vi "RegisterMessageQue.vi"(8 "error in (no error)":errorcluster, 9 "Message que":T1, 11 "SendMessage in":refnum<class "SendMessage.lvclass">) -> (0 "error out":errorcluster, 3 "SendMessage out":refnum<class "SendMessage.lvclass">)   [LabVIEW 2018, in "SendMessage.lvclass"]
uses:
  SendMessage.lvclass
  Support/MessageQue/MessageQue.ctl
  Support/MessageQue/MessageCluster.ctl
  SendMessage.lvclass/SendMessage.ctl
  Support/MessageQue/MessageQue.lvlib
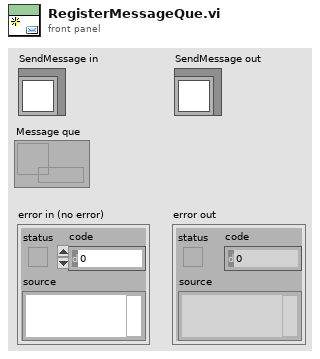
[diagram p1: front panel]
types:
  T1 = typedef "MessageQue.lvlib/MessageQue.ctl" = refnum<queue>
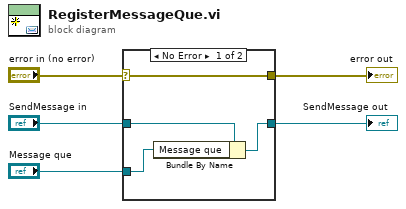
[diagram p0: block diagram]
diagram:
  n1 = case shown="No Error" "error in (no error)" {
    selector: "error in (no error)" -> [w9 w11]
    tunnel: [w9 w11] -> w4
    tunnel: [w6 w10] -> w2
    tunnel: "SendMessage in" -> [w7 w10]
    tunnel: "Message que" -> [w8 _]
    frame No Error {
      n2 = Bundle By Name(cluster=w7, "Message que"=w8) -> (w6:refnum<class "SendMessage.lvclass">)
    }
    frame Error {
    }
  }
  "error out" <- w4
  "SendMessage out" <- w2
